vi "Temperature Limit.vi"(3 "High Limit":dbl=80.0 format="%.2f", 5 "Points to Acquire":i32=75 min=20 max=500) -> ()   [LabVIEW 2010]
doc: "This VI simulates the acquisition of temperature, graphs the temperature, and notifies the user if the temperature is over the limit."
panel:
  in  "delta t (ms)":u32=400
  out "Over Limit":bool
  in  "Abort":bool
  out "Temperature":cluster{"Temperature":dbl, "High Limit":dbl}(graph)
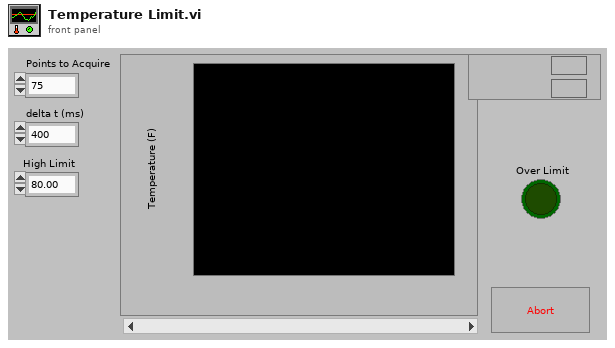
[diagram p1: front panel]
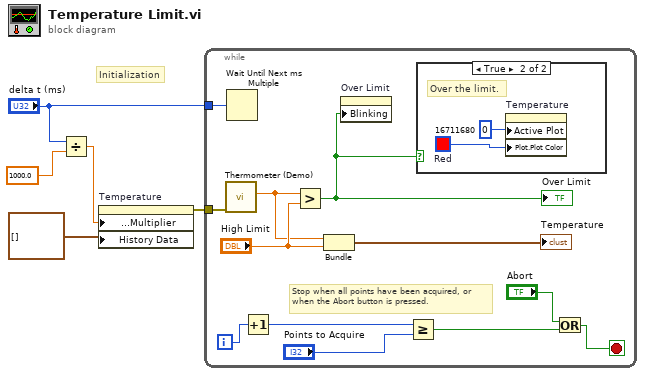
[diagram p0: block diagram]
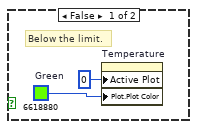
[diagram p2: hidden frame]
diagram:
  # "Initialization"
  n1 = Divide(x="delta t (ms)", y=1000.0) -> (x/y=w1:dbl)
  n2 = property on="Temperature" class="WFChart (strict)"("X Scale.Offset and Multiplier:Multiplier"=w1, "History Data"=cluster{"Temperature":dbl, "High Limit":dbl}[] []) -> (error out=w4:errorcluster)  [unwired: 2 in, 1 out]
  n3 = while {
    tunnel: "delta t (ms)" -> [w9]
    tunnel: w4 -> [w6]
    i -> [w16]
    stop <- w10 stop-if-true
    # "Stop when all points have been acquired, or when the Abort button is pressed."
    n4 = call "Thermometer (Demo).vi"("error in (no error)"=w6) -> ("Temperature"=w7:dbl)  [unwired: 8 in, 1 out]
    n5 = Wait Until Next ms Multiple(millisecond multiple=w9) -> ()  [unwired: 1 out]
    n6 = Increment(x=w16) -> (x+1=w14:i32)
    n7 = Greater?(x=w7, y="High Limit") -> (0:w8:bool)
    "Over Limit" <- w8
    n8 = Bundle("Temperature"=w7, "High Limit"="High Limit") -> (→"Temperature":cluster{"Temperature":dbl, "High Limit":dbl})  [unwired: 1 in]
    n9 = property on="Over Limit" class="Bool (strict)"("Blinking"=w8) -> ()  [unwired: 2 in, 2 out]
    n10 = Greater Or Equal?(x=w14, y="Points to Acquire") -> (x >= y?=w12:bool)
    n11 = case shown="True" w8 {
      frame False {
        w18 = u32 6618880  # Green
        # "Below the limit."
        n12 = property on="Temperature" class="WFChart (strict)"("Active Plot"=u32 0, "Plot.Plot Color"=w18) -> ()  [unwired: 2 in, 2 out]
      }
      frame True {
        w21 = u32 16711680  # Red
        # "Over the limit."
        n13 = property on="Temperature" class="WFChart (strict)"("Active Plot"=u32 0, "Plot.Plot Color"=w21) -> ()  [unwired: 2 in, 2 out]
      }
    }
    n14 = Or(x="Abort", y=w12) -> (x .or. y?=w10:bool)
  }
